vi "test_wykladniczy.vi"() -> ()   [LabVIEW 2013, in "LukiBrary.lvlib"]
uses:
  LukiBrary.lvlib
  <vilib>/Analysis/NI_AALBase.lvlib
panel:
  out "1/lambda (wartość oczekiwana)":dbl
  out "Histogram Graph":T1(graph)
  in  "lambda":dbl=1.0
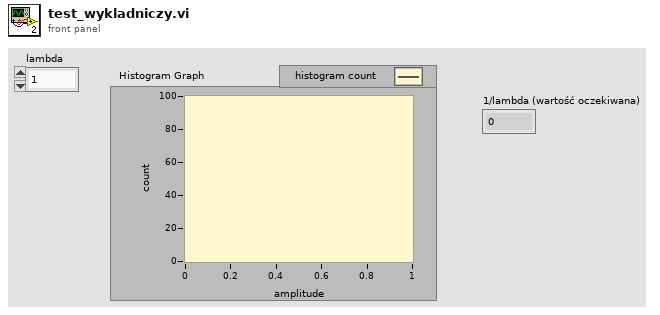
[diagram p1: front panel]
types:
  T1 = cluster{"X Values":dbl[], "Histogram: h(x)":i32[]}
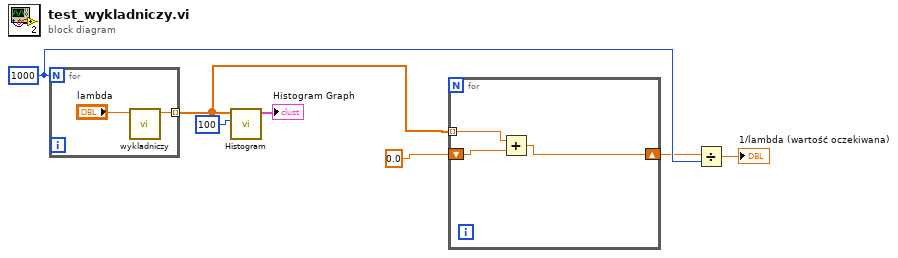
[diagram p0: block diagram]
diagram:
  w3 = 1000
  n1 = for {
    N: w3 -> [_]
    tunnel: [w8] -> w5 mode=indexing
    n2 = call "wykladniczy.vi"("lambda"="lambda") -> ("X~wykładniczy"=w8:dbl)  [unwired: 10 in]
  }
  n3 = call <vilib>:"Histogram.vi"("intervals"=100, "X"=w5) -> ("Histogram Graph"=→"Histogram Graph":T1)  [unwired: 6 in, 3 out]
  n4 = for {
    tunnel: w5 -> [w11] mode=indexing
    shift-right: [w10] -> w2
    shift-left: 0.0 -> [w12]
    n5 = Add(x=w11, y=w12) -> (x+y=w10:dbl)
  }
  n6 = Divide(x=w2, y=w3) -> (x/y=→"1/lambda (wartość oczekiwana)":dbl)
